vi "Parse Arguments.vi"(8 "error in (no error)":errorcluster, 10 "Inputs":string[](array[string]), 11 "LUnitCLI In":refnum<class "LUnitCLI.lvclass">) -> (0 "error out":errorcluster, 3 "LUnitCLI Out":refnum<class "LUnitCLI.lvclass">)   [LabVIEW 2020, in "LUnitCLI.lvclass"]
uses:
  LUnitCLI.lvclass
  LUnitCLI.lvclass/LUnitCLI.ctl
  <vilib>/ErrorRing/Error Ring.xnode
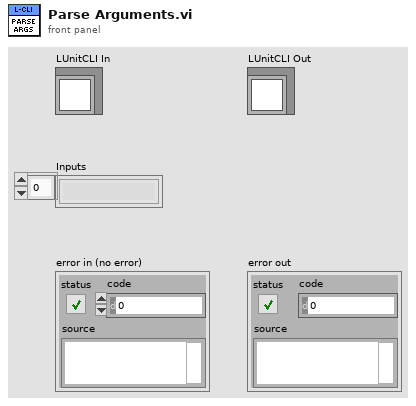
[diagram p1: front panel]
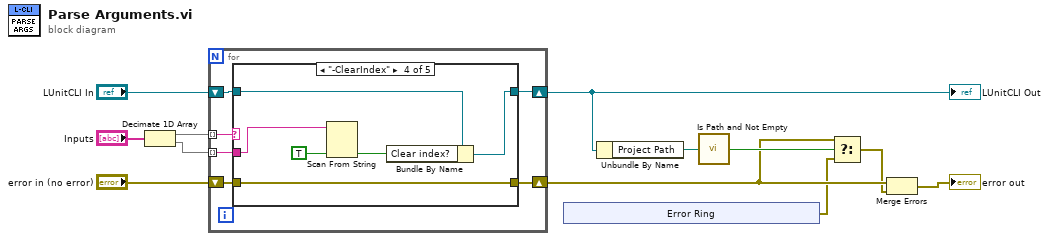
[diagram p0: block diagram]
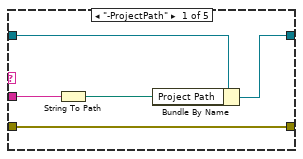
[diagram p2: hidden frame]
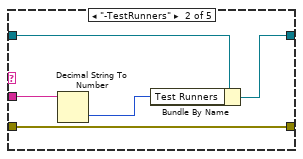
[diagram p3: hidden frame]
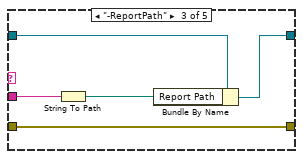
[diagram p4: hidden frame]
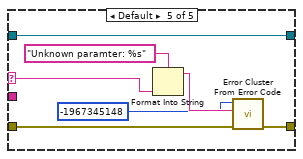
[diagram p5: hidden frame]
diagram:
  n1 = Decimate 1D Array("Inputs") -> (w9:string[], w10:string[])
  n2 = for {
    tunnel: w9 -> [w18] mode=indexing
    tunnel: w10 -> [w17] mode=indexing
    shift-right: [w15] -> w7
    shift-left: "LUnitCLI In" -> [w16]
    shift-right: [w14] -> w3
    shift-left: "error in (no error)" -> [w13]
    n3 = case shown="\"-ClearIndex\"" w18 {
      selector: w18 -> [_ _ _ _ w45]
      tunnel: w17 -> [w20 w24 w30 w36 _]
      tunnel: w16 -> [w23 w28 w33 w39 w40]
      tunnel: [w22 w27 w32 w38 w40] -> w15
      tunnel: [w21 w26 w31 w37 w44] -> w14
      tunnel: w13 -> [w21 w26 w31 w37 w41]
      frame "-ProjectPath" {
        n4 = String To Path(string=w20) -> (path=w19:path)
        n5 = Bundle By Name(cluster=w23, "Project Path"=w19) -> (w22:refnum<class "LUnitCLI.lvclass">)
      }
      frame "-TestRunners" {
        n6 = Decimal String To Number(string=w24) -> (number=w25:i32)  [unwired: 2 in, 1 out]
        n7 = Bundle By Name(cluster=w28, "Test Runners"=w25) -> (w27:refnum<class "LUnitCLI.lvclass">)
      }
      frame "-ReportPath" {
        n8 = String To Path(string=w30) -> (path=w29:path)
        n9 = Bundle By Name(cluster=w33, "Report Path"=w29) -> (w32:refnum<class "LUnitCLI.lvclass">)
      }
      frame "-ClearIndex" {
        n10 = Scan From String(input string=w36, default 1=TRUE) -> (output 1=w35:bool)  [unwired: 3 in, 3 out]
        n11 = Bundle By Name(cluster=w39, "Clear index?"=w35) -> (w38:refnum<class "LUnitCLI.lvclass">)
      }
      frame Default {
        n12 = Format Into String(format string="Unknown paramter: %s", w45) -> (resulting string=w43:string)  [unwired: 2 in, 1 out]
        n13 = call <vilib>:"Error Cluster From Error Code.vi"("error in (no error)"=w41, "error message (\"\")"=w43, "error code (0)"=-1967345148) -> ("error out"=w44:errorcluster)  [unwired: 6 in]
      }
    }
  }
  "LUnitCLI Out" <- w7
  n14 = xnode "Error Ring"() -> ("error out"=w2:errorcluster)
  n15 = Unbundle By Name(w7) -> ("Project Path"=w6:path)
  n16 = call <vilib>:"Is Path and Not Empty.vi"("path"=w6) -> ("Is Path and Not Empty?"=w4:bool)  [unwired: 4 in]
  n17 = Select(t=w3, s=w4, f=w2) -> (s? t:f=w1:errorcluster)
  n18 = Merge Errors(w3, w1) -> (→"error out":errorcluster)
